vi "PB_add_VLIW.vi"(0 "VLIW Array In":T1(array[cluster]) {"OP Code" format="%.0x"; "Output Bits" format="%.0x"}, 1 "Data Field":u32, 2 "Digital Bits":u32 format="%.0x", 3 "Delay":dbl=50.0 format="%.3p", 4 "OP code":u8(ring) items=["Continue", "Stop", "Loop", "End Loop", "Jump", "Return", "Go To", "Long Delay"], 5 "error in (no error)":errorcluster) -> (6 "VLIW Array Out":T1(array[cluster])=[{"Output Bits"=0, "Data Field"=3, "OP Code"=2, "Delay Count"=4}, {"Output Bits"=0, "Data Field"=0, "OP Code"=3, "Delay Count"=4}, {"Output Bits"=0, "Data Field"=0, "OP Code"=0, "Delay Count"=2599999997}, {"Output Bits"=0, "Data Field"=2, "OP Code"=7, "Delay Count"=1073741821}, {"Output Bits"=0, "Data Field"=0, "OP Code"=0, "Delay Count"=705032701}] {"OP Code" format="%.0x"; "Output Bits" format="%.0x"}, 7 "Actual Delay":dbl=50.0 format="%.2p", 8 "error out":errorcluster)   [LabVIEW 2013]
doc: "This vi writes a single command to \"VLIW Array\", where \"VLIW array\" is an array of clusters which contain an image of the command array of the PulseBlaster.\n\nIt provides some error checking on the inputs to help make sure you won't confuse the PulseBlaster.\nInputs:\n 1) Digital Bits (24 bit output flags)\n 2) Data Field (24 bits)\n 3) OP Code (4 bits)\n 4) Delay (in units of seconds)\n 5) error in.\n 6) Input array (The array to be appended to.)\nOutputs\n 1) Actual Delay (in units of seconds, rounded to nearest 10ns)\n 2) error out.\n 3) Output array. (The appended array.)\n\n\"PB_add_VLIW\" uses the globally defined variables in \"PB_defines\". The long delay command should be entirely transparent, so the user does not need to envoke it."
uses:
  PB_defines.vi
panel:
  # "append"
  # "to"
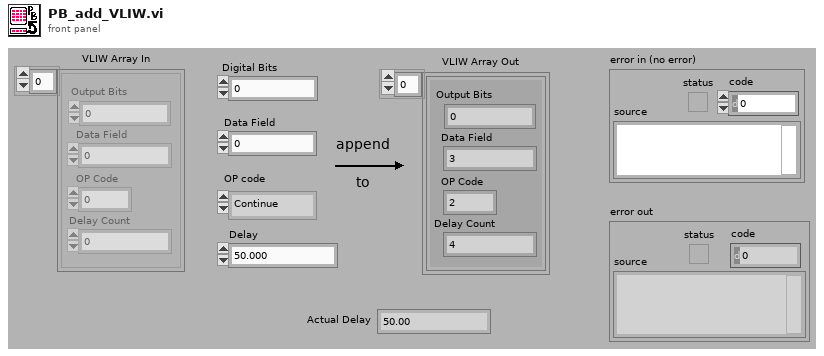
[diagram p1: front panel]
types:
  T1 = cluster{"Output Bits":u32, "Data Field":u32, "OP Code":u8, "Delay Count":u32}[]
  T2 = cluster{"Output Bits":u32, "Data Field":u32, "OP Code":u8, "Delay Count":u32}
  T3 = cluster{"Digital Bits":u32, "Data Field":u32, "OP code":i32, u32}
  T4 = cluster{"Digital Bits":u32, u32, "OP code":i32, u32}
  T5 = cluster{"Digital Bits":u32, "Data Field":u32, "OP code":i32, "Delay Count":u32}[]
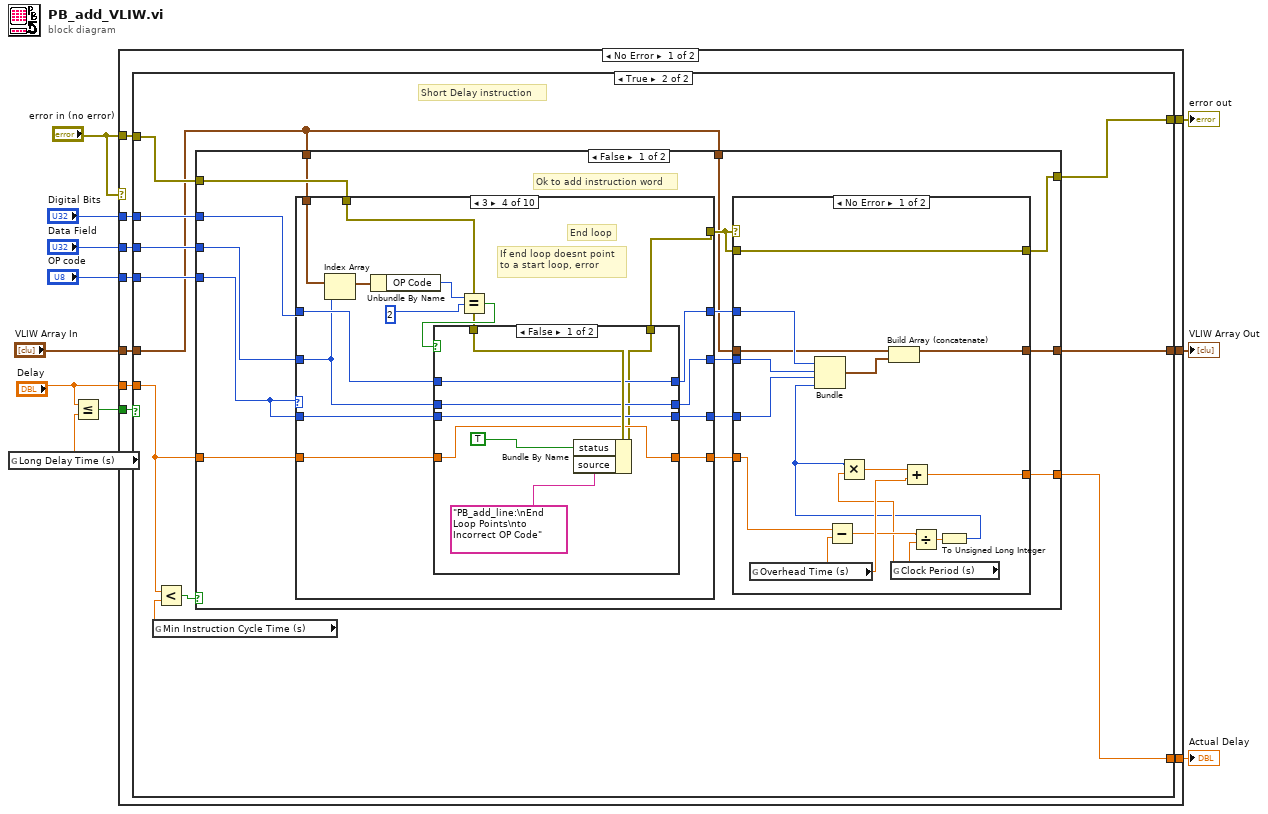
[diagram p0: block diagram]
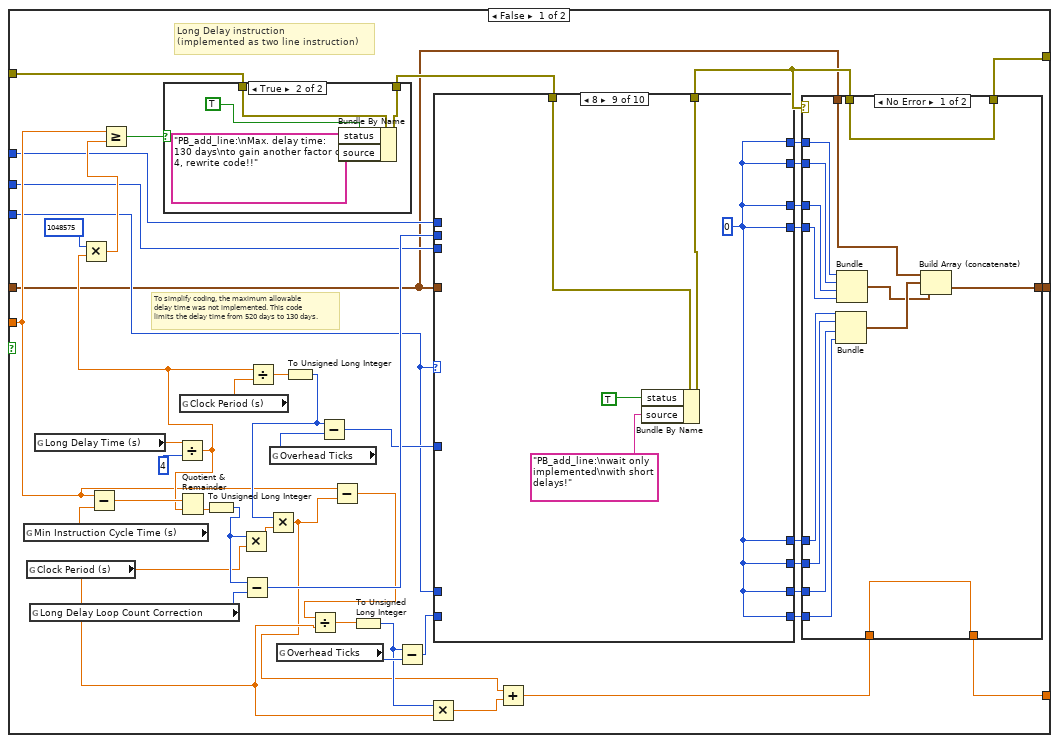
[diagram p2: hidden frame]
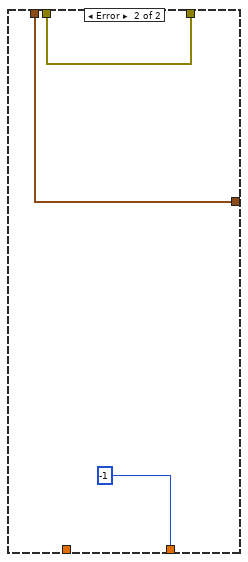
[diagram p4: hidden frame]
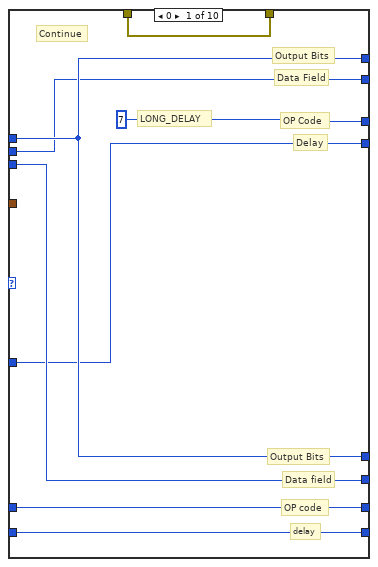
[diagram p5: hidden frame]
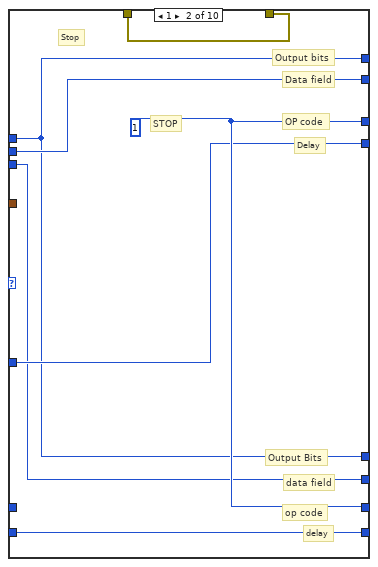
[diagram p6: hidden frame]
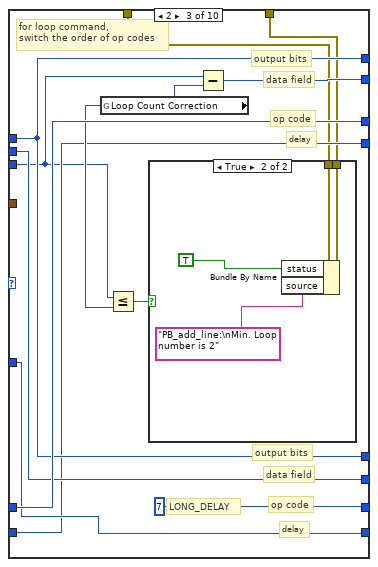
[diagram p7: hidden frame]
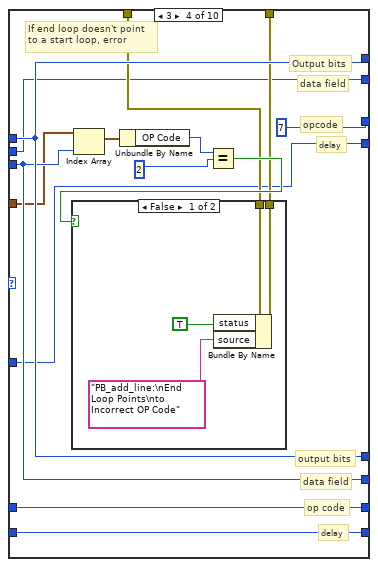
[diagram p9: hidden frame]
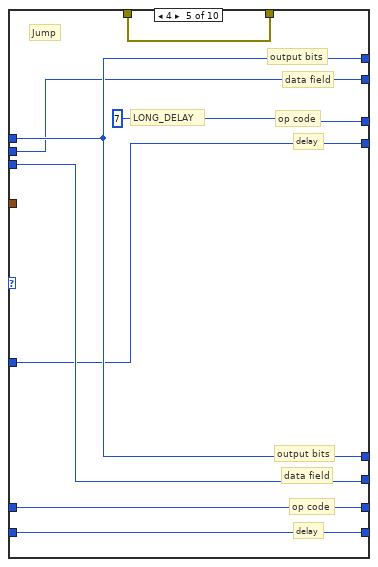
[diagram p11: hidden frame]
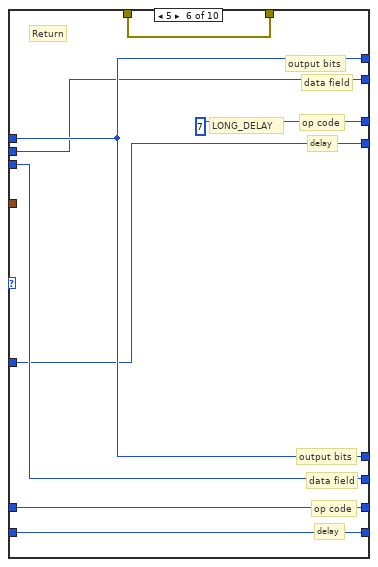
[diagram p12: hidden frame]
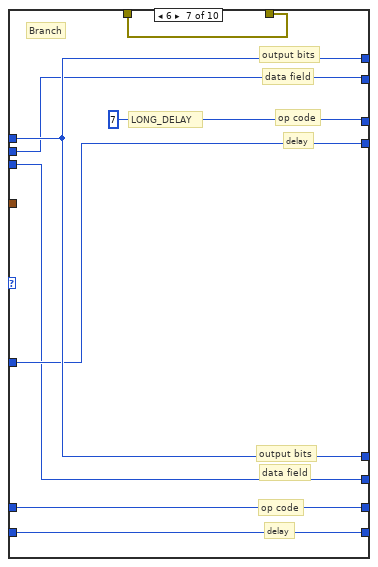
[diagram p13: hidden frame]
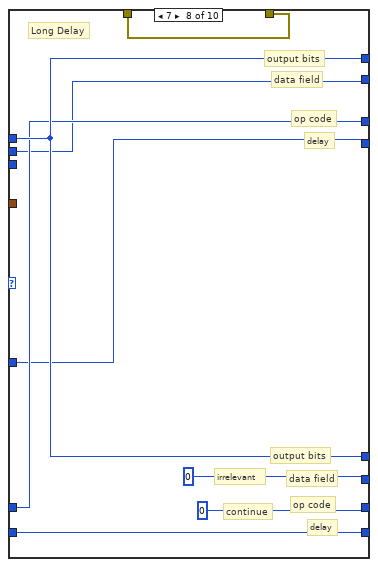
[diagram p14: hidden frame]
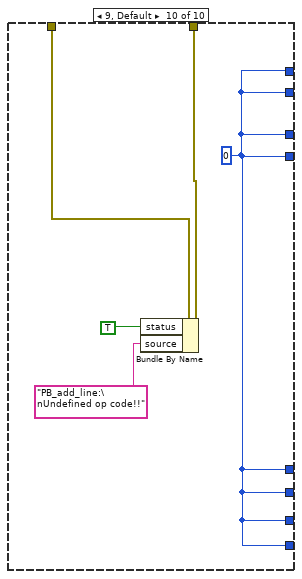
[diagram p15: hidden frame]
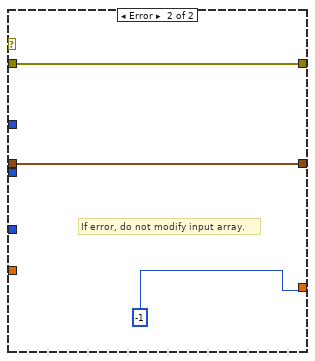
[diagram p16: hidden frame]
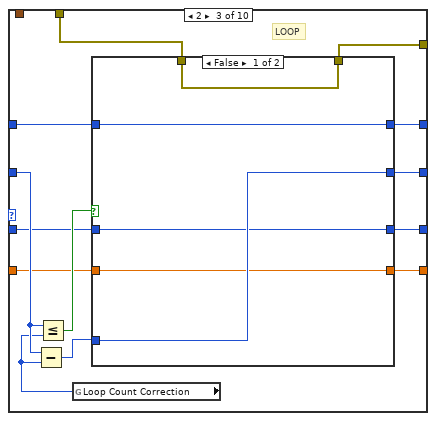
[diagram p19: hidden frame]
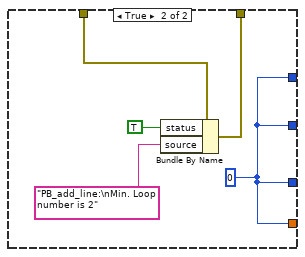
[diagram p20: hidden frame]
diagram:
  n1 = global read "PB_defines.vi" "Long Delay Time (s)"() -> (w11:dbl)
  n2 = Less Or Equal?(x="Delay", y=w11) -> (x <= y?=w10:bool)
  n3 = case shown="No Error" "error in (no error)" {
    tunnel: w10 -> [w21 _]
    tunnel: "error in (no error)" -> [w20 w331]
    tunnel: [w19 w331] -> w9
    tunnel: [w18 -1] -> w7
    tunnel: "Delay" -> [w17 _]
    tunnel: [w16 w329] -> w6
    tunnel: "VLIW Array In" -> [w15 w329]
    tunnel: "Digital Bits" -> [w14 _]
    tunnel: "Data Field" -> [w13 _]
    tunnel: "OP code" -> [w12 _]
    frame No Error {
      n4 = case shown="True" w21 {
        tunnel: w20 -> [w31 w191]
        tunnel: [w49 w190] -> w19
        tunnel: [w27 w189] -> w18
        tunnel: w17 -> [w29 w188]
        tunnel: [w23 w187] -> w16
        tunnel: w15 -> [w22 w183]
        tunnel: w14 -> [w26 w186]
        tunnel: w13 -> [w25 w185]
        tunnel: w12 -> [w24 w184]
        frame False {
          # "To simplify coding, the maximum allowable\ndelay time was not implemented. This code \nlimits the delay time from 520 days to 130 days."
          # "Long Delay instruction \n(implemented as two line instruction)"
          n5 = global read "PB_defines.vi" "Min Instruction Cycle Time (s)"() -> (w66:dbl)
          n6 = global read "PB_defines.vi" "Clock Period (s)"() -> (w39:dbl)
          n7 = global read "PB_defines.vi" "Long Delay Loop Count Correction"() -> (w64:u8)
          n8 = global read "PB_defines.vi" "Long Delay Time (s)"() -> (w36:dbl)
          n9 = Subtract(x=w29, y=w66) -> (x-y=w65:dbl)
          n10 = Divide(x=w36, y=4) -> (x/y=w34:dbl)
          n11 = Multiply(x=1048575, y=w34) -> (x*y=w33:dbl)
          n12 = Greater Or Equal?(x=w29, y=w33) -> (x >= y?=w32:bool)
          n13 = case shown="True" w32 {
            tunnel: w31 -> [w68 w70]
            tunnel: [w68 w69] -> w30
            frame False {
            }
            frame True {
              n14 = Bundle By Name(cluster=w70, "status"=TRUE, "source"="PB_add_line:\nMax. delay time: 130 days\nto gain another factor of 4, rewrite code!!") -> (w69:errorcluster)
            }
          }
          n15 = Quotient & Remainder(x=w65, y=w34) -> (floor(x/y)=w41:dbl)  [unwired: 1 out]
          n16 = global read "PB_defines.vi" "Clock Period (s)"() -> (w48:dbl)
          n17 = To Unsigned Long Integer(number=w41) -> (unsigned 32bit integer=w40:u32)
          n18 = Multiply(x=w40, y=w39) -> (x*y=w62:dbl)
          n19 = Subtract(x=w40, y=w64) -> (x-y=w63:u32)
          n20 = Divide(x=w34, y=w48) -> (x/y=w47:dbl)
          n21 = global read "PB_defines.vi" "Overhead Ticks"() -> (w45:u8)
          n22 = global read "PB_defines.vi" "Overhead Ticks"() -> (w44:u8)
          n23 = To Unsigned Long Integer(number=w47) -> (unsigned 32bit integer=w46:u32)
          n24 = Multiply(x=w46, y=w62) -> (x*y=w37:dbl)
          n25 = Subtract(x=w46, y=w45) -> (x-y=w60:u32)
          n26 = Subtract(x=w29, y=w37) -> (x-y=w43:dbl)
          n27 = Divide(x=w43, y=w39) -> (x/y=w61:dbl)
          n28 = To Unsigned Long Integer(number=w61) -> (unsigned 32bit integer=w42:u32)
          n29 = Subtract(x=w42, y=w44) -> (x-y=w50:u32)
          n30 = Multiply(x=w42, y=w39) -> (x*y=w38:dbl)
          n31 = case shown="8" w24 {
            tunnel: w24 -> [w94 _ w115 w134 w146 w154 w162 w169 _ _]
            tunnel: [7 w104 w115 7 7 7 7 w169 w173 w178] -> w54
            tunnel: [w94 w104 7 w134 w146 w154 w162 0 w173 w178] -> w57
            tunnel: [w95 w99 w114 w125 w143 w151 w157 0 w173 w178] -> w58
            tunnel: w26 -> [w97 w98 w111 w135 w147 w155 w163 w172 _ _]
            tunnel: [w97 w98 w111 w135 w147 w155 w163 w172 w173 w178] -> w52
            tunnel: [w97 w98 w111 w135 w147 w155 w163 w172 w173 w178] -> w59
            tunnel: w60 -> [w90 w102 w110 w123 w142 w149 w158 w167 _ _]
            tunnel: [w90 w102 w109 w123 w142 w149 w158 w167 w173 w178] -> w55
            tunnel: [w96 w103 w112 w126 w141 w152 w160 w166 w173 w178] -> w53
            tunnel: w63 -> [w96 w103 w114 w126 w141 w152 w160 w166 _ _]
            tunnel: w25 -> [w95 w99 w107 w125 w143 w151 w157 _ _ _]
            tunnel: [w93 w101 w110 w124 w144 w150 w159 w170 w173 w178] -> w56
            tunnel: w50 -> [w93 w101 w109 w124 w144 w150 w159 w170 _ _]
            tunnel: w30 -> [w92 w100 w106 w129 w145 w153 w161 w171 w175 w180]
            tunnel: [w92 w100 w105 w128 w145 w153 w161 w171 w174 w179] -> w51
            tunnel: w22 -> [_ _ _ w122 _ _ _ _ _ _]
            frame 0 {
              # "Continue"
              # "delay"
              # "OP code"
              # "Data field"
              # "Output Bits"
              # "Delay"
              # "Data Field"
              # "OP Code"
              # "Output Bits"
              # "LONG_DELAY"
            }
            frame 1 {
              w104 = 1
              # "Stop"
              # "delay"
              # "op code"
              # "data field"
              # "Output Bits"
              # "Delay"
              # "OP code"
              # "Data field"
              # "Output bits"
              # "STOP"
            }
            frame 2 {
              # "for loop command,\nswitch the order of op codes"
              # "delay"
              # "op code"
              # "data field"
              # "output bits"
              # "delay"
              # "op code"
              # "data field"
              # "output bits"
              # "LONG_DELAY"
              n32 = global read "PB_defines.vi" "Loop Count Correction"() -> (w113:u8)
              n33 = Less Or Equal?(x=w107, y=w113) -> (x <= y?=w108:bool)
              n34 = case shown="True" w108 {
                tunnel: w106 -> [w117 w119]
                tunnel: [w117 w118] -> w105
                frame False {
                }
                frame True {
                  n35 = Bundle By Name(cluster=w119, "status"=TRUE, "source"="PB_add_line:\nMin. Loop number is 2") -> (w118:errorcluster)
                }
              }
              n36 = Subtract(x=w107, y=w113) -> (x-y=w112:u32)
            }
            frame 3 {
              # "delay"
              # "op code"
              # "data field"
              # "output bits"
              # "delay"
              # "opcode"
              # "data field"
              # "Output bits"
              # "If end loop doesn't point\nto a start loop, error"
              n37 = Index Array(array=w122, index=w125) -> (element=w131:T2)
              n38 = Unbundle By Name(w131) -> ("OP Code"=w130:u8)
              n39 = Equal?(x=w130, y=2) -> (x = y?=w132:bool)
              n40 = case shown="False" w132 {
                tunnel: [w138 w140] -> w128
                tunnel: w129 -> [w137 w140]
                frame False {
                  n41 = Bundle By Name(cluster=w137, "status"=TRUE, "source"="PB_add_line:\nEnd Loop Points\nto Incorrect OP Code") -> (w138:errorcluster)
                }
                frame True {
                }
              }
            }
            frame 4 {
              # "Jump"
              # "data field"
              # "delay"
              # "delay"
              # "op code"
              # "data field"
              # "output bits"
              # "output bits"
              # "op code"
              # "LONG_DELAY"
            }
            frame 5 {
              # "Return"
              # "delay"
              # "op code"
              # "data field"
              # "output bits"
              # "delay"
              # "op code"
              # "data field"
              # "output bits"
              # "LONG_DELAY"
            }
            frame 6 {
              # "Branch"
              # "delay"
              # "op code"
              # "data field"
              # "output bits"
              # "delay"
              # "op code"
              # "data field"
              # "output bits"
              # "LONG_DELAY"
            }
            frame 7 {
              # "Long Delay"
              # "irrelevant"
              # "continue"
              # "delay"
              # "op code"
              # "data field"
              # "output bits"
              # "delay"
              # "op code"
              # "data field"
              # "output bits"
            }
            frame 8 {
              w173 = 0
              n42 = Bundle By Name(cluster=w175, "status"=TRUE, "source"="PB_add_line:\nwait only implemented\nwith short delays!") -> (w174:errorcluster)
            }
            frame 9, Default {
              w178 = 0
              n43 = Bundle By Name(cluster=w180, "status"=TRUE, "source"="PB_add_line:\nUndefined op code!!") -> (w179:errorcluster)
            }
          }
          n44 = Add(x=w37, y=w38) -> (x+y=w28:dbl)
          n45 = case shown="No Error" w51 {
            tunnel: w59 -> [w86 _]
            tunnel: w58 -> [w85 _]
            tunnel: w57 -> [w84 _]
            tunnel: w56 -> [w83 _]
            tunnel: w55 -> [w82 _]
            tunnel: w54 -> [w81 _]
            tunnel: w53 -> [w80 _]
            tunnel: w52 -> [w79 _]
            tunnel: [w78 w89] -> w49
            tunnel: w51 -> [w78 w89]
            tunnel: [w77 -1] -> w27
            tunnel: w28 -> [w77 _]
            tunnel: [w76 w87] -> w23
            tunnel: w22 -> [w75 w87]
            frame No Error {
              n46 = Bundle("Digital Bits"=w86, "Data Field"=w85, "OP code"=w84, w83) -> (w74:T3)  [unwired: 1 in]
              n47 = Bundle("Digital Bits"=w79, w80, "OP code"=w81, w82) -> (w73:T4)  [unwired: 1 in]
              n48 = Build Array (concatenate)(w75, w74, w73) -> (w76:T5)
            }
            frame Error {
            }
          }
        }
        frame True {
          # "Short Delay instruction"
          n49 = global read "PB_defines.vi" "Min Instruction Cycle Time (s)"() -> (w193:dbl)
          n50 = Less?(x=w188, y=w193) -> (x < y?=w192:bool)
          n51 = case shown="False" w192 {
            tunnel: w191 -> [w208 w328]
            tunnel: [w207 w327] -> w190
            tunnel: [w201 -1] -> w189
            tunnel: w188 -> [w200 _]
            tunnel: [w199 w324] -> w187
            tunnel: w183 -> [w198 w324]
            tunnel: w186 -> [w197 _]
            tunnel: w185 -> [w196 _]
            tunnel: w184 -> [w195 _]
            tunnel: w183 -> [w194 _]
            frame False {
              # "Ok to add instruction word"
              n52 = case shown="3" w195 {
                tunnel: w208 -> [w231 w232 w246 w271 w292 w293 w298 w309 w317 w319]
                tunnel: [w231 w232 w245 w272 w292 w293 w298 w308 w317 w320] -> w202
                tunnel: [w230 w236 w244 w266 w291 w297 w302 w307 w316 w318] -> w206
                tunnel: w197 -> [w230 w236 w240 w270 w291 w297 w302 w307 w316 _]
                tunnel: [w229 w235 w243 w265 w290 w296 w301 w306 w315 w318] -> w205
                tunnel: w196 -> [w229 w235 w249 w269 w290 w296 w301 w306 w315 _]
                tunnel: [w228 w234 w242 w264 w289 w295 w300 w305 w314 w318] -> w204
                tunnel: w195 -> [w228 w234 w238 w268 w289 w295 w300 w305 w314 _]
                tunnel: [w227 w233 w241 w263 w288 w294 w299 w304 w311 w318] -> w203
                tunnel: w200 -> [w227 w233 w239 w267 w288 w294 w299 w304 w312 _]
                tunnel: w194 -> [_ _ _ w260 _ _ _ _ _ _]
                frame 0 {
                  # "Continue"
                }
                frame 1 {
                  # "Stop"
                }
                frame 2 {
                  # "LOOP"
                  n53 = global read "PB_defines.vi" "Loop Count Correction"() -> (w248:u8)
                  n54 = Subtract(x=w249, y=w248) -> (x-y=w237:u32)
                  n55 = Less Or Equal?(x=w249, y=w248) -> (x <= y?=w247:bool)
                  n56 = case shown="False" w247 {
                    tunnel: w246 -> [w254 w257]
                    tunnel: [w254 w256] -> w245
                    tunnel: [w253 w255] -> w244
                    tunnel: [w252 w255] -> w243
                    tunnel: [w250 w255] -> w242
                    tunnel: [w251 w255] -> w241
                    tunnel: w240 -> [w253 _]
                    tunnel: w237 -> [w252 _]
                    tunnel: w239 -> [w251 _]
                    tunnel: w238 -> [w250 _]
                    frame False {
                    }
                    frame True {
                      w255 = 0
                      n57 = Bundle By Name(cluster=w257, "status"=TRUE, "source"="PB_add_line:\nMin. Loop number is 2") -> (w256:errorcluster)
                    }
                  }
                }
                frame 3 {
                  # "If end loop doesnt point\nto a start loop, error"
                  # "End loop"
                  n58 = Index Array(array=w260, index=w269) -> (element=w262:T2)
                  n59 = Unbundle By Name(w262) -> ("OP Code"=w261:u8)
                  n60 = Equal?(x=w261, y=2) -> (x = y?=w273:bool)
                  n61 = case shown="False" w273 {
                    tunnel: [w275 w287] -> w272
                    tunnel: w271 -> [w280 w287]
                    tunnel: w270 -> [w277 w285]
                    tunnel: w269 -> [w279 w284]
                    tunnel: [w279 w284] -> w265
                    tunnel: w268 -> [w276 w283]
                    tunnel: w267 -> [w278 w286]
                    tunnel: [w278 w286] -> w263
                    tunnel: [w277 w285] -> w266
                    tunnel: [w276 w283] -> w264
                    frame False {
                      n62 = Bundle By Name(cluster=w280, "status"=TRUE, "source"="PB_add_line:\nEnd Loop Points\nto Incorrect OP Code") -> (w275:errorcluster)
                    }
                    frame True {
                    }
                  }
                }
                frame 4 {
                }
                frame 5 {
                }
                frame 6 {
                }
                frame 7 {
                  n63 = Bundle By Name(cluster=w309, "status"=TRUE, "source"="PB_add_line:\nLong delay op code requires\ndelay to be larger than 42.949 s") -> (w308:errorcluster)
                }
                frame 8 {
                  # "WAIT op code has 6 clock\ncycle overhead, rather than\nusual 3 cycles, so subtract\noff an additional 30 ns."
                  n64 = Subtract(x=w312, y=3e-08) -> (x-y=w311:dbl)
                }
                frame 9, Default {
                  w318 = 0
                  n65 = Bundle By Name(cluster=w319, "status"=TRUE, "source"="PB_add_line:\nUndefined op code.") -> (w320:errorcluster)
                }
              }
              n66 = case shown="No Error" w202 {
                tunnel: [w223 w226] -> w207
                tunnel: w202 -> [w223 w226]
                tunnel: w206 -> [w215 _]
                tunnel: w205 -> [w216 _]
                tunnel: w204 -> [w217 _]
                tunnel: w203 -> [w218 _]
                tunnel: [w211 -1] -> w201
                tunnel: [w210 w224] -> w199
                tunnel: w198 -> [w209 w224]
                frame No Error {
                  n67 = global read "PB_defines.vi" "Overhead Time (s)"() -> (w222:dbl)
                  n68 = Subtract(x=w218, y=w222) -> (x-y=w221:dbl)
                  n69 = global read "PB_defines.vi" "Clock Period (s)"() -> (w220:dbl)
                  n70 = Divide(x=w221, y=w220) -> (x/y=w219:dbl)
                  n71 = To Unsigned Long Integer(number=w219) -> (unsigned 32bit integer=w213:u32)
                  n72 = Bundle("Digital Bits"=w215, "Data Field"=w216, "OP code"=w217, w213) -> (w214:T3)  [unwired: 1 in]
                  n73 = Multiply(x=w213, y=w220) -> (x*y=w212:dbl)
                  n74 = Build Array (concatenate)(w209, w214) -> (w210:T5)
                  n75 = Add(x=w212, y=w222) -> (x+y=w211:dbl)
                }
                frame Error {
                  # "If error, do not modify input array."
                }
              }
            }
            frame True {
              # "error"
              n76 = Bundle By Name(cluster=w328, "status"=TRUE, "source"="PB_add_line:\nDelay Time too short") -> (w327:errorcluster)
            }
          }
        }
      }
    }
    frame Error {
      # "If an error occurs, don't modify the input array."
    }
  }
  "error out" <- w9
  "Actual Delay" <- w7
  "VLIW Array Out" <- w6
